vi "Generate_Sinewave.vi"(8 "error in (no error)":errorcluster, 9 "cycles":dbl=500.0 format="%#_13g", 10 "samples":i32=5000) -> (0 "error out":errorcluster, 1 "Power Spectrum":dbl[](graph), 3 "Data String":string)   [LabVIEW 2019, in "Sending_larger_data.lvlib"]
uses:
  Sending_larger_data.lvlib
  <vilib>/Analysis/2dsp.llb/Power Spectrum (DBL).vi
  <vilib>/Analysis/NI_AALBase.lvlib
  <vilib>/Analysis/NI_AALPro.lvlib
panel:
  out "Messages":string
  out "Data (kB)":dbl
  out "interleaved array":i16[](array[numeric])
  out "Signal Time domain":dbl[](graph)
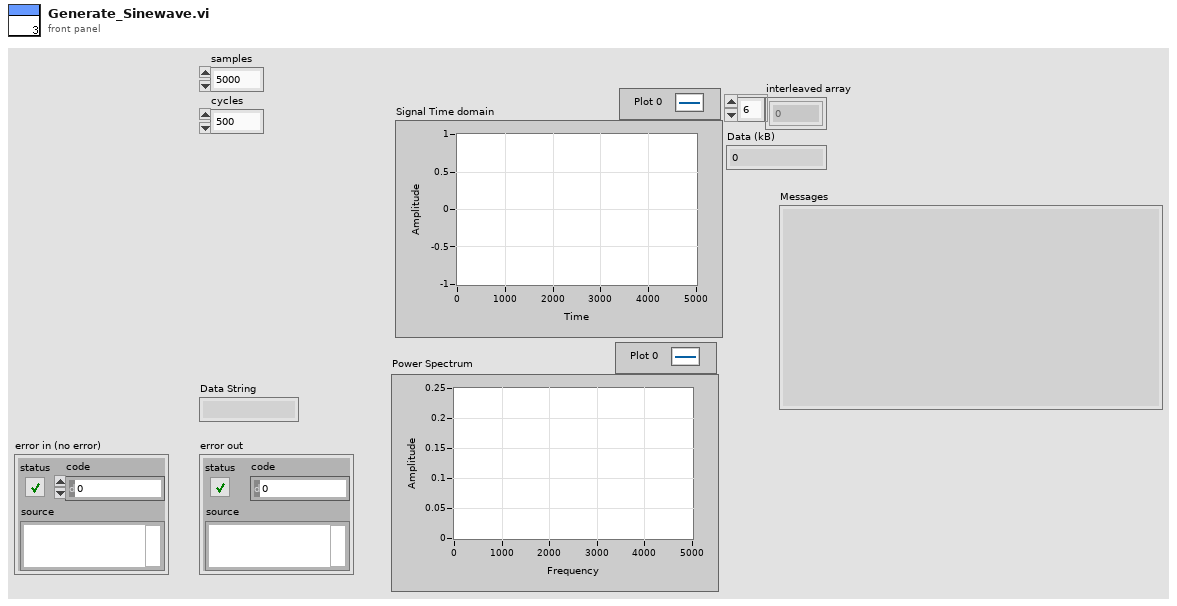
[diagram p1: front panel]
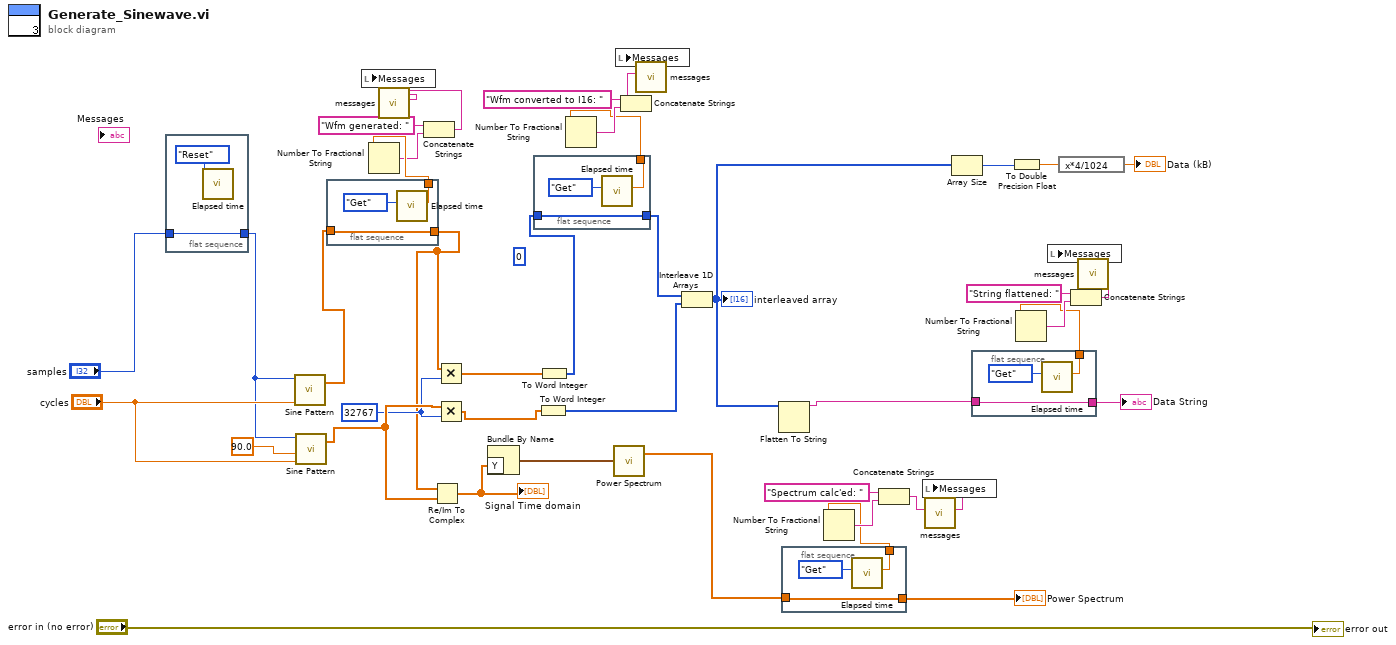
[diagram p0: block diagram]
diagram:
  w39 = i16 32767
  (unwired) i16 0
  n1 = flat-sequence {
    tunnel: "samples" -> [w45]
    tunnel: [w45] -> w30
    frame #0 {
      n2 = call "Elapsed time.vi"("Mode"=enum16{"Get", "Reset"}."Reset") -> ()  [unwired: 8 in, 3 out]
    }
  }
  n3 = call <vilib>:"Sine Pattern.vi"("cycles"="cycles", "samples"=w30) -> ("Sinusoidal Pattern"=w5:dbl[])  [unwired: 2 in, 1 out]
  n4 = call <vilib>:"Sine Pattern.vi"("cycles"="cycles", "phase(degrees)"=90.0, "samples"=w30) -> ("Sinusoidal Pattern"=w40:dbl[])  [unwired: 1 in, 1 out]
  n5 = flat-sequence {
    tunnel: [w48] -> w4
    tunnel: w5 -> [w48]
    tunnel: [w47] -> w8
    frame #0 {
      n6 = call "Elapsed time.vi"("Mode"=enum16{"Get", "Reset"}."Get") -> ("Elapsed sec"=w47:dbl)  [unwired: 8 in, 2 out]
    }
  }
  n7 = Number To Fractional String(number=w8) -> (F-format string=w7:string)  [unwired: 3 in]
  n8 = Concatenate Strings("Wfm generated: " ("string"), w7) -> (w3:string)
  n9 = call "messages.vi"("Message"=w3) -> ("Messages"=w2:string)  [unwired: 9 in, 1 out]
  n10 = local write "Messages"(w2) -> ()
  n11 = Re/Im To Complex(1:w40, 2:w4) -> (0:w41:cdb[])
  "Signal Time domain" <- w41
  n12 = Multiply(x=w4, y=w39) -> (x*y=w38:dbl[])
  n13 = Multiply(x=w40, y=w39) -> (x*y=w37:dbl[])
  n14 = Bundle By Name("Y"=w41) -> (w12:waveform(cdb))  [unwired: 1 in]
  n15 = flat-sequence {
    tunnel: [w51] -> w28
    tunnel: w29 -> [w51]
    tunnel: [w50] -> w22
    frame #0 {
      n16 = call "Elapsed time.vi"("Mode"=enum16{"Get", "Reset"}."Get") -> ("Elapsed sec"=w50:dbl)  [unwired: 8 in, 2 out]
    }
  }
  n17 = To Word Integer(number=w37) -> (16bit integer=w36:i16[])
  n18 = To Word Integer(number=w38) -> (16bit integer=w29:i16[])
  n19 = Number To Fractional String(number=w22) -> (F-format string=w23:string)  [unwired: 3 in]
  n20 = call-poly <vilib>:"Power Spectrum.vi"("X"=w12) -> ("Power Spectrum"=w11:dbl[])  [unwired: 1 out]
  n21 = Concatenate Strings("Wfm converted to I16: " ("string"), w23) -> (w25:string)
  n22 = call "messages.vi"("Message"=w25) -> ("Messages"=w18:string)  [unwired: 9 in, 1 out]
  n23 = local write "Messages"(w18) -> ()
  n24 = Interleave 1D Arrays(w28, w36) -> (w32:i16[])
  "interleaved array" <- w32
  n25 = Flatten To String(anything=w32) -> (data string=w27:string)  [unwired: 3 in, 2 out]
  n26 = flat-sequence {
    tunnel: [w54] -> w10
    tunnel: w11 -> [w54]
    tunnel: [w53] -> w9
    frame #0 {
      n27 = call "Elapsed time.vi"("Mode"=enum16{"Get", "Reset"}."Get") -> ("Elapsed sec"=w53:dbl)  [unwired: 8 in, 2 out]
    }
  }
  n28 = Number To Fractional String(number=w9) -> (F-format string=w13:string)  [unwired: 3 in]
  n29 = Concatenate Strings("Spectrum calc'ed: " ("string"), w13) -> (w15:string)
  n30 = call "messages.vi"("Message"=w15) -> ("Messages"=w1:string)  [unwired: 9 in, 1 out]
  n31 = local write "Messages"(w1) -> ()
  n32 = Array Size(array=w32) -> (size(s)=w35:i32)
  n33 = flat-sequence {
    tunnel: [w57] -> w26
    tunnel: w27 -> [w57]
    tunnel: [w56] -> w16
    frame #0 {
      n34 = call "Elapsed time.vi"("Mode"=enum16{"Get", "Reset"}."Get") -> ("Elapsed sec"=w56:dbl)  [unwired: 8 in, 2 out]
    }
  }
  n35 = To Double Precision Float(number=w35) -> (double precision float=w34:dbl)
  n36 = Number To Fractional String(number=w16) -> (F-format string=w21:string)  [unwired: 3 in]
  n37 = expression code="x*4/1024"(w34) -> (→"Data (kB)":dbl)
  n38 = Concatenate Strings("String flattened: " ("string"), w21) -> (w19:string)
  n39 = call "messages.vi"("Message"=w19) -> ("Messages"=w17:string)  [unwired: 9 in, 1 out]
  n40 = local write "Messages"(w17) -> ()
  "error out" <- "error in (no error)"
  "Data String" <- w26
  "Power Spectrum" <- w10
